vi "FX55.vi"(11 "Variables and Memory in":T1 {"GFX" format="%02x"}) -> (3 "Variables and Memory out":T1 {"GFX" format="%02x"})   [LabVIEW 2021]
uses:
  Controls/ClusterF.ctl
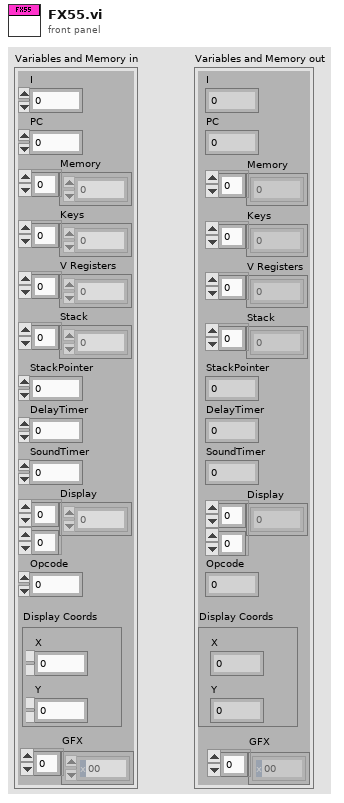
[diagram p1: front panel]
types:
  T1 = typedef "ClusterF.ctl" = cluster{"I":u16, "PC":u16, "Memory":u8[], "Keys":u8[], "V Registers":u8[], "Stack":u16[], "StackPointer":u16, "DelayTimer":u8, "SoundTimer":u8, "Display":u8[][], "Opcode":u16, "Display Coords":cluster{"X":u8, "Y":u8}, "GFX":u8[]}
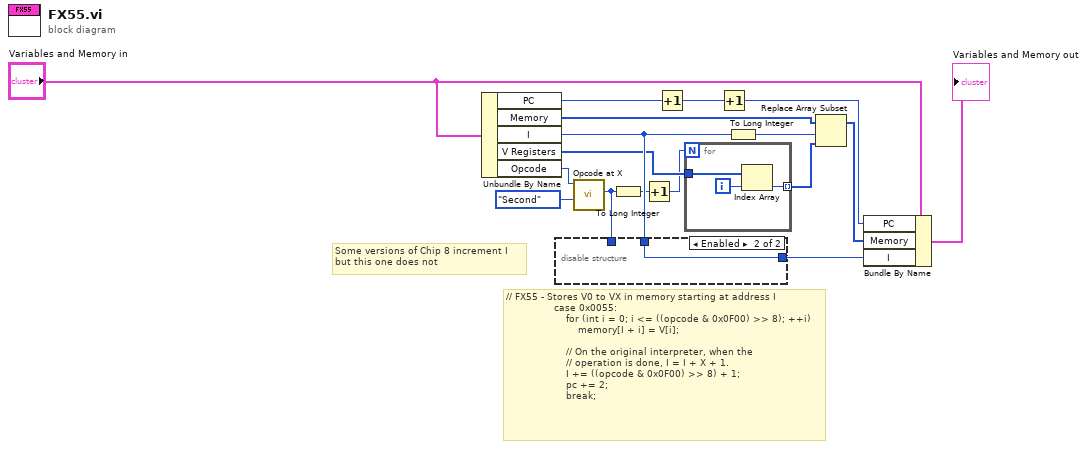
[diagram p0: block diagram]
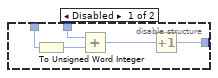
[diagram p2: hidden frame]
diagram:
  # "Some versions of Chip 8 increment I\nbut this one does not"
  # "// FX55 - Stores V0 to VX in memory starting at address I\n                case 0x0055:\n                    for (int i = 0; i <= ((opcode & 0x0F00) >> 8); ++i)\n                        memory[I + i] = V[i];\n\n                    // On the original interpreter, when the\n                    // operation is done, I = I + X + 1.\n                    I += ((opcode & 0x0F00) >> 8) + 1;\n                    pc += 2;\n                    break;"
  n1 = Unbundle By Name("Variables and Memory in") -> ("PC"=w4:u16, "Memory"=w9:u8[], "I"=w15:u16, "V Registers"=w12:u8[], "Opcode"=w8:u16)
  n2 = call "Opcode at X.vi"("X Position"=enum16{"First", "Second", "Third", "Fourth"}."Second", "Opcode"=w8) -> ("Opcode at X Position (U8)"=w16:u8)  [unwired: 9 in]
  n3 = disable-structure shown="Enabled" {
    disable-tunnel: [w22 w23] -> w17
    disable-tunnel: w16 -> [w19 _]
    disable-tunnel: w15 -> [w18 w23]
    frame Disabled {
      n4 = To Unsigned Word Integer(number=w19) -> (unsigned 16bit integer=w20:u16)
      n5 = Add(x=w18, y=w20) -> (x+y=w21:u16)
      n6 = Increment(x=w21) -> (x+1=w22:u16)
    }
    frame Enabled {
    }
  }
  n7 = To Long Integer(number=w16) -> (32bit integer=w11:i32)
  n8 = Increment(x=w11) -> (x+1=w1:i32)
  n9 = Increment(x=w4) -> (x+1=w5:u16)
  n10 = for {
    N: w1 -> [_]
    tunnel: w12 -> [w26]
    tunnel: [w25] -> w13 mode=indexing
    i -> [w24]
    n11 = Index Array(array=w26, index=w24) -> (element=w25:u8)
  }
  n12 = Increment(x=w5) -> (x+1=w6:u16)
  n13 = To Long Integer(number=w15) -> (32bit integer=w10:i32)
  n14 = Replace Array Subset(array=w9, new element=w13, index=w10) -> (w14:u8[])
  n15 = Bundle By Name(cluster="Variables and Memory in", "PC"=w6, "Memory"=w14, "I"=w17) -> (→"Variables and Memory out":T1)
